vi "GOLPI Initialize.vi"(7 "processing setup":T1={"mode"=enum."Raw", "call after avgs?"=FALSE, "calculate?"=FALSE, "raw mode"={"command"="", "result mode"=enum."Display console output (only Octave)", "res variable"=""}, "QWTB"={"QWTB path"=path "", "alg filter path"="", "alg ids"=[], "alg parameters"=[], "parsed parameters"=[], "selected alg id"="", "selected unc mode"=enum."None", "qwtb mcc"=100, "qwtb timeout"=90, "qwtb covg"=95.0, "qwtb ofs"=0, "qwtb lim data"=0, "multicore"={"jobs folder"=path "", "cores"=0, "max jobs"=0, "mode"=enum."Singlecore"}, "unc once?"=FALSE}}, 8 "error in":errorcluster, 10 "Start Octave? (False)":bool, 11 "golpi session ref":T10) -> (0 "error out":errorcluster, 2 "GNU Octave version":string, 3 "golpi session out (copy)":T10)   [LabVIEW 2013]
doc: "Call this somewhere on startup of the application. It will initialize GOLPI Multi Process lib, i.e. GOLPI wrapper for safe use of the GOLPI in multi-process/thread applications where GOLPI may be accessed from multiple VIs simultaneously. \nIt will setup initial and exit commands. These are command sequences that will be executed whenever Octave is started or before exit. These are typically used to store current environemnt to disk and restore it when application starts again. Optionally it may start Octave. Otherwise it will be started automatically when used for the first time."
uses:
  golpi_session_ref.ctl
  golpi_session.ctl
  GOLPI Library.lvlibp/Public/GOLPI reference Type Def.ctl
  GOLPI Library.lvlibp/LV Process source distribution/Pipe Handle.ctl
  measure/processing/Meas Process Config.ctl
  measure/processing/Meas Process Mode.ctl
  measure/processing/Meas Process Raw Config.ctl
  measure/processing/Meas Process Raw Result Mode.ctl
  measure/processing/QWTB/Meas Proc QWTB Setup.ctl
  measure/processing/QWTB/Meas Proc QWTB Algorithm Parameter Data.ctl
  measure/processing/QWTB/Meas Proc QWTB Uncertainty Mode.ctl
  measure/processing/QWTB/Meas Proc QWTB Multicore Setup.ctl
  measure/processing/QWTB/Meas Proc QWTB Multicore Type.ctl
  GOLPI Multi Process.lvlib
  GOLPI Library.lvlibp/LV Process source distribution/LV Process library.lvlib
  GOLPI Library.lvlibp
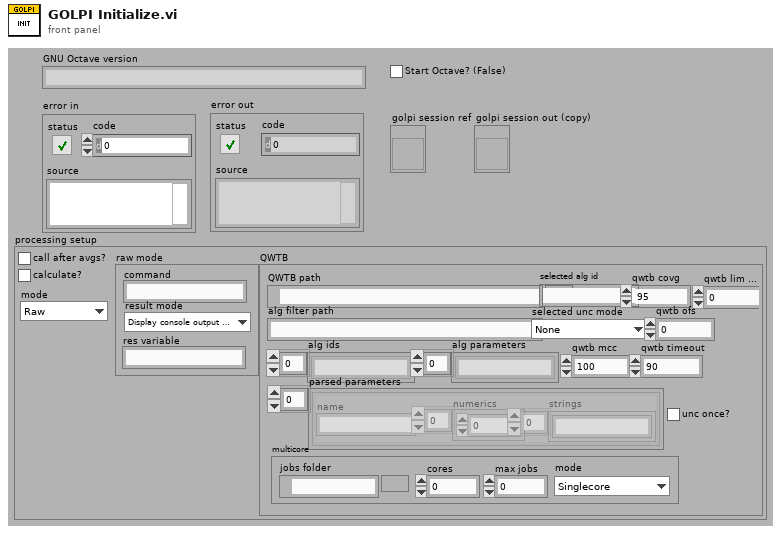
[diagram p1: front panel]
types:
  T1 = typedef "Meas Process Config.ctl" = cluster{"mode":T2, "call after avgs?":bool, "calculate?":bool, "raw mode":T3, "QWTB":T5}
  T2 = typedef "Meas Process Mode.ctl" = enum16{"Raw", "QWTB"}
  T3 = typedef "Meas Process Raw Config.ctl" = cluster{"command":string, "result mode":T4, "res variable":string}
  T4 = typedef "Meas Process Raw Result Mode.ctl" = enum16{"Display console output (only Octave)", "Display string variable", "Display result file %respath%"}
  T5 = typedef "Meas Proc QWTB Setup.ctl" = cluster{"QWTB path":path, "alg filter path":string, "alg ids":string[], "alg parameters":string[], "parsed parameters":T6[], "selected alg id":string, "selected unc mode":T7, "qwtb mcc":i32, "qwtb timeout":i32, "qwtb covg":dbl, "qwtb ofs":i64, "qwtb lim data":i64, "multicore":T8, "unc once?":bool}
  T6 = typedef "Meas Proc QWTB Algorithm Parameter Data.ctl" = cluster{"name":string, "numerics":dbl[], "strings":string[]}
  T7 = typedef "Meas Proc QWTB Uncertainty Mode.ctl" = enum16{"None", "GUF", "Monte Carlo"}
  T8 = typedef "Meas Proc QWTB Multicore Setup.ctl" = cluster{"jobs folder":path, "cores":i32, "max jobs":i32, "mode":T9}
  T9 = typedef "Meas Proc QWTB Multicore Type.ctl" = enum16{"Singlecore", "Multicore", "Multistation"}
  T10 = typedef "GOLPI Multi Process.lvlib/golpi_session_ref.ctl" = refnum<vi>
  T11 = typedef "GOLPI Library.lvlibp/GOLPI reference Type Def.ctl" = cluster{"pipe handle":T12, "fast read timeout [ms]":u32, "fast read settle time [ms]":u32, "fast read to multiple [ms]":u32, "max elements per input line":u32, "slow read timeout [ms]":u32, "stdin double format specifier":string, "max elements per stdout output column":u32, "console mode bitstream":bool, "bitstream first read timeout [ms]":u32, "bitstream read timeout [ms]":u32, "struct transfer possible":bool, "matlab mode":bool}
  T12 = typedef "GOLPI Library.lvlibp/LV Process library.lvlib/Pipe Handle.ctl" = cluster{"lv_proc.dll file path":path, "process instance handle":u32[], "debug mode":bool, "debug data":cluster{"time":timestamp, "stdin":bool, "data":string}[]}
  T13 = typedef "GOLPI Multi Process.lvlib/golpi_session.ctl" = cluster{"GOLPI ref":T11, "idn str":string, "octave path":path, "work path":path, "start timeout [ms]":u32, "clr cache":bool, "console":bool, "binary":bool, "semaphore":T14, "initial command":string, "exit command":string, "matlab":bool}
  T14 = typedef "Semaphore RefNum" = refnum<k1>
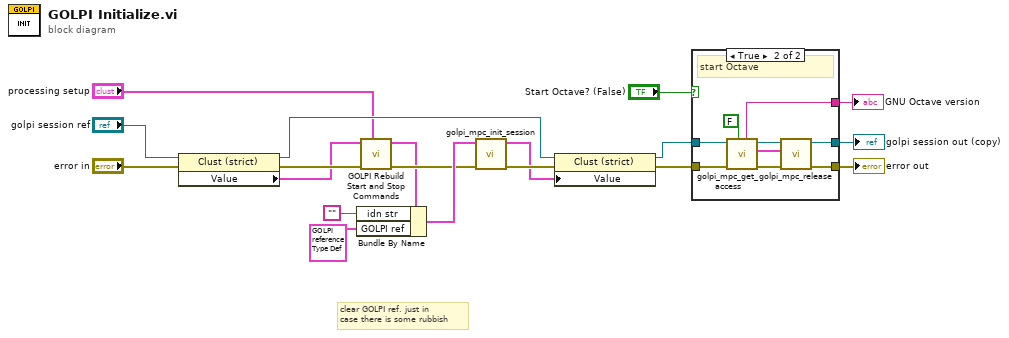
[diagram p0: block diagram]
diagram:
  # "clear GOLPI ref. just in\ncase there is some rubbish"
  n1 = property class="Clust (strict)"(reference="golpi session ref", error in="error in") -> (reference out=w13:T10, error out=w5:errorcluster, "Value"=w2:T13)
  n2 = call "GOLPI Rebuild Start and Stop Commands.vi"("processing setup"="processing setup", "error in"=w5, "golpi session in"=w2) -> ("error out"=w4:errorcluster, "golpi session out"=w3:T13)  [unwired: 7 in]
  n3 = Bundle By Name(cluster=w3, "idn str"="", "GOLPI ref"=T11 {"pipe handle"={"lv_proc.dll file path"=path "", "process instance handle"=[], "debug mode"=FALSE, "debug data"=[]}, "fast read timeout [ms]"=500, "fast read settle time [ms]"=10, "fast read to multiple [ms]"=1, "max elements per input line"=100, "slow read timeout [ms]"=5000, "stdin double format specifier"="%_16e", "max elements per stdout output column"=100, "console mode bitstream"=FALSE, "bitstream first read timeout [ms]"=1000, "bitstream read timeout [ms]"=50, "struct transfer possible"=FALSE, "matlab mode"=FALSE}) -> (w16:T13)
  n4 = call "golpi_mpc_init_session.vi"("error in"=w4, "golpi session in"=w16) -> ("error out"=w15:errorcluster, "golpi session out"=w14:T13)  [unwired: 8 in]
  n5 = property class="Clust (strict)"(reference=w13, error in=w15, "Value"=w14) -> (reference out=w11:T10, error out=w12:errorcluster)
  n6 = case shown="True" "Start Octave? (False)" {
    tunnel: w12 -> [w20 w30]
    tunnel: w11 -> [w21 w27]
    tunnel: [w20 w26] -> w10
    tunnel: [w21 w23] -> w9
    tunnel: [_ w22] -> w8
    frame False {
    }
    frame True {
      # "start Octave"
      n7 = call "golpi_mpc_get_access.vi"("don't query version (true)"=FALSE, "error in"=w30, "golpi session ref"=w27) -> ("error out"=w29:errorcluster, "golpi session out"=w25:T13, "golpi session ref out (copy)"=w28:T10, "GNU Octave version"=w22:string)  [unwired: 3 in, 2 out]
      n8 = call "golpi_mpc_release.vi"("error in"=w29, "golpi ref or golpi session in"=w25, "golpi session ref"=w28) -> ("error out"=w26:errorcluster, "golpi session out (copy)"=w23:T10)  [unwired: 7 in]
    }
  }
  "error out" <- w10
  "golpi session out (copy)" <- w9
  "GNU Octave version" <- w8
